vi "Teleop.vi"(10 "Match Info":T1={"Autonomous Elapsed Seconds"=0.0, "TeleOp Elapsed Seconds"=0.0, "Disabled Elapsed Seconds"=0.0, "Visited Autonomous"=FALSE, "Visited TeleOp"=FALSE, "Visited Disabled"=FALSE, "Autonomous Settings"={"Autonomous Style"=enum."Independent", "VI Refnum"=refnum}}, 11 "Call Context":T2) -> ()   [LabVIEW 2014]
doc: "This VI is called for each TeleOp packet received from the DS where the robot is not disabled. It is often used to read from the joysticks and update I/O or to update setpoints for timed control loops. It should complete and return within 20 milliseconds or it may miss DS packets."
uses:
  <vilib>/Rock Robotics/WPI/DriverStation/WPI_DriverStationDerivedRobotMode.ctl
  <vilib>/Rock Robotics/WPI/DriverStation/WPI_DriverStationMatch Info.ctl
  <vilib>/Rock Robotics/Network Tables/SD Read Boolean.vi
  <vilib>/Rock Robotics/Network Tables/SD Read Number.vi
  <vilib>/Rock Robotics/WPI/Joystick/WPI_JoystickGetSetRefNum.vi
  Robot Global Data.vi
panel:
  out "Sample Slider 0":dbl(slide) scale=0.0..5.0
  out "Sample Boolean 1":bool
  out "Sample Boolean 0":bool
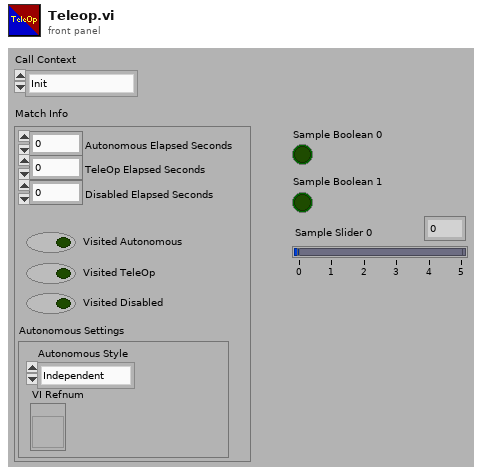
[diagram p1: front panel]
types:
  T1 = typedef "WPI_DriverStationMatch Info.ctl" = cluster{"Autonomous Elapsed Seconds":dbl, "TeleOp Elapsed Seconds":dbl, "Disabled Elapsed Seconds":dbl, "Visited Autonomous":bool, "Visited TeleOp":bool, "Visited Disabled":bool, "Autonomous Settings":cluster{"Autonomous Style":enum16{"Iterative", "Independent"}, "VI Refnum":refnum<vi>}}
  T2 = typedef "WPI_DriverStationDerivedRobotMode.ctl" = enum16{"Init", "Execute", "Stop"}
  T3 = typedef "WPI_JoystickDevRef.ctl" = cluster{"Device":T4}
  T4 = typedef "WPI_JoystickDeviceEnum.ctl" = enum16{"USB 0", "USB 1", "USB 2", "USB 3", "USB 4", "USB 5"}
  T5 = cluster{"Button 1":bool, "Button 2":bool, "Button 3":bool, "Button 4":bool, "Button 5":bool, "Button 6":bool, "Button 7":bool, "Button 8":bool, "Button 9":bool, "Button 10":bool, "Button 11":bool, "Button 12":bool}
  T6 = cluster{"axis 1 (x)":dbl, "axis 2 (y)":dbl, "axis 3 (throttle)":dbl, "axis 4":dbl, "axis 5":dbl, "axis 6":dbl}
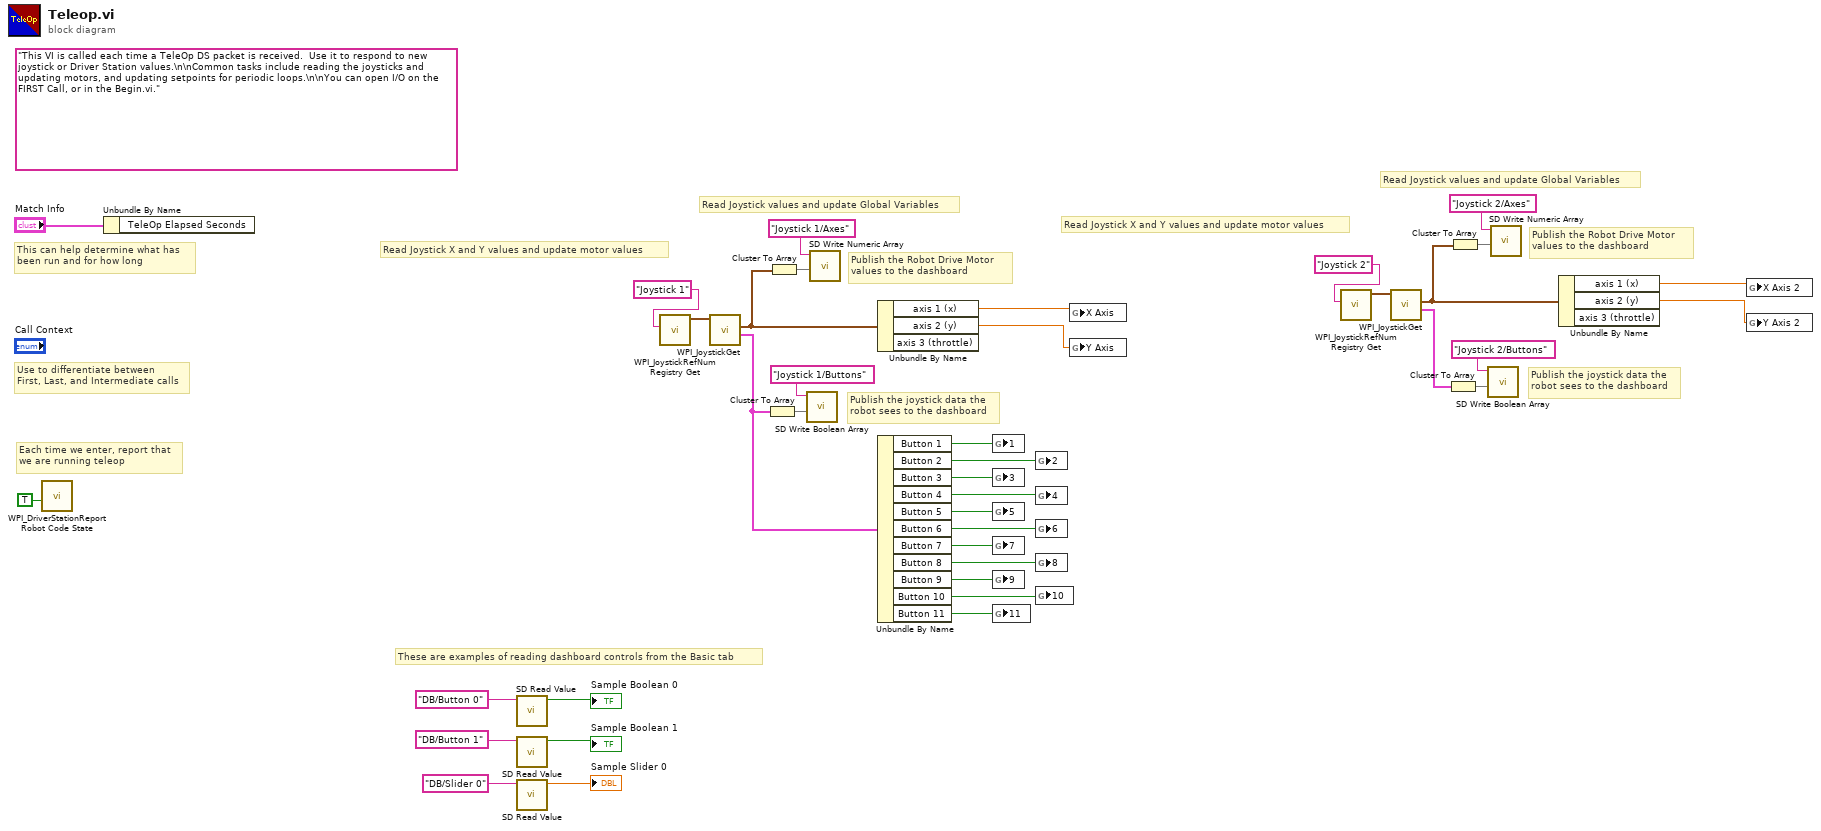
[diagram p0: block diagram]
diagram:
  (unwired) "This VI is called each time a TeleOp DS packet is received.  Use it to respond to new joystick or Driver Station values.\n\nCommon tasks include reading the joysticks and updating motors, and updating setpoints for periodic loops.\n\nYou can open I/O on the FIRST Call, or in the Begin.vi."
  # "Publish the Robot Drive Motor\nvalues to the dashboard"
  # "Publish the joystick data the\nrobot sees to the dashboard"
  # "Read Joystick values and update Global Variables"
  # "Read Joystick X and Y values and update motor values"
  # "Publish the Robot Drive Motor\nvalues to the dashboard"
  # "Publish the joystick data the\nrobot sees to the dashboard"
  # "Read Joystick values and update Global Variables"
  # "These are examples of reading dashboard controls from the Basic tab"
  # "Each time we enter, report that\nwe are running teleop"
  # "Use to differentiate between\nFirst, Last, and Intermediate calls"
  # "This can help determine what has\nbeen run and for how long"
  # "Read Joystick X and Y values and update motor values"
  n1 = call <vilib>:"WPI_DriverStationReport Robot Code State.vi"("TeleOp"=TRUE ("Autonomous")) -> ()  [unwired: 10 in, 1 out]
  n2 = Unbundle By Name("Match Info") -> ()  [unwired: 1 out]
  n3 = call-poly <vilib>:"SD Read Value.vi"("Name"="DB/Button 0" ("refnum name")) -> ("Boolean"=→"Sample Boolean 0":bool)  [unwired: 8 in, 2 out]
  n4 = call-poly <vilib>:"SD Read Value.vi"("Name"="DB/Button 1" ("refnum name")) -> ("Boolean"=→"Sample Boolean 1":bool)  [unwired: 8 in, 2 out]
  n5 = call-poly <vilib>:"SD Read Value.vi"("Name"="DB/Slider 0" ("refnum name")) -> ("Numeric"=→"Sample Slider 0":dbl)  [unwired: 8 in, 2 out]
  n6 = call <vilib>:"WPI_JoystickRefNum Registry Get.vi"("refnum name"="Joystick 1") -> ("JoystickDevRef"=w31:T3)  [unwired: 1 in, 9 out]
  n7 = call <vilib>:"WPI_JoystickGet.vi"("JoystickDevRef"=w31) -> ("Buttons"=w25:T5, "Axes"=w28:T6)  [unwired: 1 in, 4 out]
  n8 = Cluster To Array(cluster=w25) -> (array=w30:bool[])
  n9 = Cluster To Array(cluster=w28) -> (array=w27:dbl[])
  n10 = call <vilib>:"SD Write Boolean Array.vi"("Boolean Array"=w30, "Name"="Joystick 1/Buttons") -> ()  [unwired: 8 in, 2 out]
  n11 = call <vilib>:"SD Write Numeric Array.vi"("Numeric Array"=w27, "Name"="Joystick 1/Axes") -> ()  [unwired: 8 in, 2 out]
  n12 = Unbundle By Name(w28) -> ("axis 1 (x)"=w13:dbl, "axis 2 (y)"=w12:dbl)  [unwired: 1 out]
  n13 = Unbundle By Name(w25) -> ("Button 1"=w24:bool, "Button 2"=w22:bool, "Button 3"=w21:bool, "Button 4"=w20:bool, "Button 5"=w19:bool, "Button 6"=w23:bool, "Button 7"=w18:bool, "Button 8"=w17:bool, "Button 9"=w16:bool, "Button 10"=w15:bool, "Button 11"=w14:bool)
  n14 = global write "Robot Global Data.vi" "1"(w24) -> ()
  n15 = global write "Robot Global Data.vi" "3"(w21) -> ()
  n16 = global write "Robot Global Data.vi" "5"(w19) -> ()
  n17 = global write "Robot Global Data.vi" "7"(w18) -> ()
  n18 = global write "Robot Global Data.vi" "9"(w16) -> ()
  n19 = global write "Robot Global Data.vi" "11"(w14) -> ()
  n20 = global write "Robot Global Data.vi" "2"(w22) -> ()
  n21 = global write "Robot Global Data.vi" "4"(w20) -> ()
  n22 = global write "Robot Global Data.vi" "6"(w23) -> ()
  n23 = global write "Robot Global Data.vi" "8"(w17) -> ()
  n24 = global write "Robot Global Data.vi" "10"(w15) -> ()
  n25 = global write "Robot Global Data.vi" "X Axis"(w13) -> ()
  n26 = global write "Robot Global Data.vi" "Y Axis"(w12) -> ()
  n27 = call <vilib>:"WPI_JoystickRefNum Registry Get.vi"("refnum name"="Joystick 2") -> ("JoystickDevRef"=w10:T3)  [unwired: 1 in, 9 out]
  n28 = call <vilib>:"WPI_JoystickGet.vi"("JoystickDevRef"=w10) -> ("Buttons"=w4:T5, "Axes"=w7:T6)  [unwired: 1 in, 4 out]
  n29 = Cluster To Array(cluster=w4) -> (array=w9:bool[])
  n30 = Cluster To Array(cluster=w7) -> (array=w6:dbl[])
  n31 = call <vilib>:"SD Write Boolean Array.vi"("Boolean Array"=w9, "Name"="Joystick 2/Buttons") -> ()  [unwired: 8 in, 2 out]
  n32 = call <vilib>:"SD Write Numeric Array.vi"("Numeric Array"=w6, "Name"="Joystick 2/Axes") -> ()  [unwired: 8 in, 2 out]
  n33 = Unbundle By Name(w7) -> ("axis 1 (x)"=w3:dbl, "axis 2 (y)"=w2:dbl)  [unwired: 1 out]
  n34 = global write "Robot Global Data.vi" "X Axis 2"(w3) -> ()
  n35 = global write "Robot Global Data.vi" "Y Axis 2"(w2) -> ()
